vi "Polling_EX.vi"() -> ()   [LabVIEW 2021]
uses:
  <vilib>/Utility/miscctls.llb/LVPoint32TypeDef.ctl
panel:
  out "Coords":T1
  out "Current Time":timestamp
  in  "Time Check":bool
  out "Iteration":i32
  in  "Stop":bool
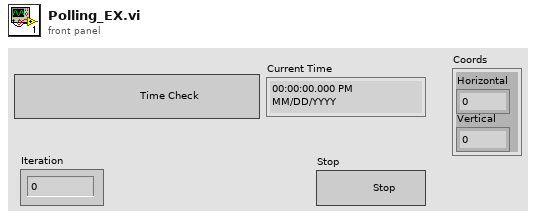
[diagram p1: front panel]
types:
  T1 = typedef "LVPoint32TypeDef.ctl" = cluster{"Horizontal":i32, "Vertical":i32}
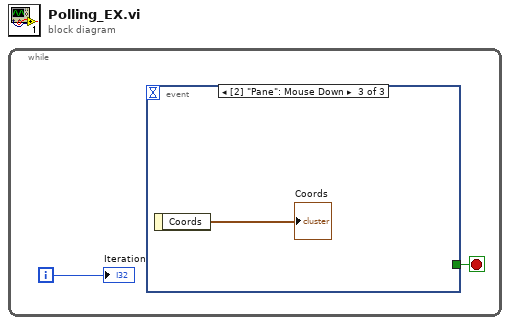
[diagram p0: block diagram]
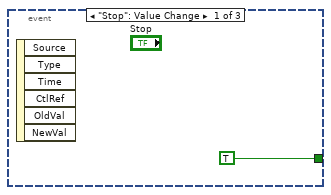
[diagram p2: hidden frame]
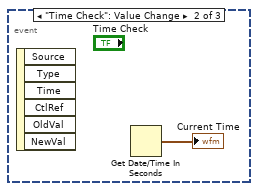
[diagram p3: hidden frame]
diagram:
  n1 = while {
    i -> [w2]
    stop <- w1 stop-if-true
    n2 = event shown="[2] \"Pane\": Mouse Down" {
      selector: _ -> [_ _ _]
      dyn-events: _ -> [_ _ _]
      timeout: _ -> [_ _ _]
      tunnel: [TRUE _ _] -> w1
      event "Stop": Value Change {
        n3 = event-data() -> ()  [unwired: 1 in, 6 out]
      }
      event "Time Check": Value Change {
        n4 = event-data() -> ()  [unwired: 1 in, 6 out]
        n5 = Get Date/Time In Seconds() -> (seconds since 1Jan1904=→"Current Time":timestamp)
      }
      event Mouse Down {
        n6 = event-data() -> ("Coords"=→"Coords":T1)  [unwired: 1 in]
      }
    }
    "Iteration" <- w2
  }
